vi "CleanGraph.vi"(9 "Bin Size":i32, 10 "N Sigma":dbl=4.0 format="%#_13g", 11 "XY Graph In":cluster{dbl[], dbl[]}(graph)) -> (3 "XY Graph Out":cluster{dbl[], dbl[]}(graph))   [LabVIEW 2019]
panel:
  in  "Repeat Until Clean (F: Run Once)":bool
  out "Smoothed":cluster{dbl[], dbl[]}(graph)
  out "Cleaned":cluster{dbl[], dbl[]}(graph)
  out "Ordered":cluster{dbl[], dbl[]}(graph)
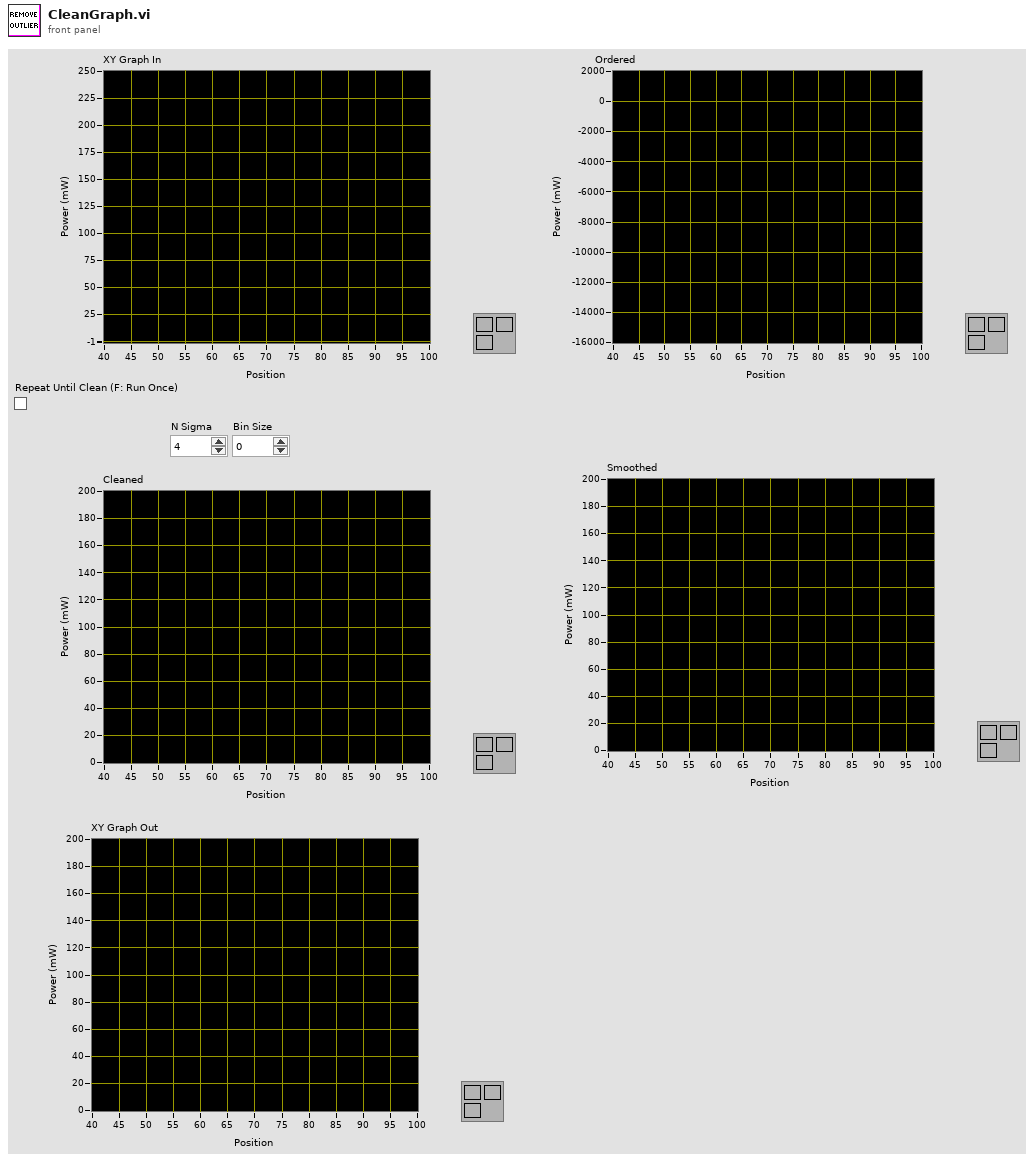
[diagram p1: front panel]
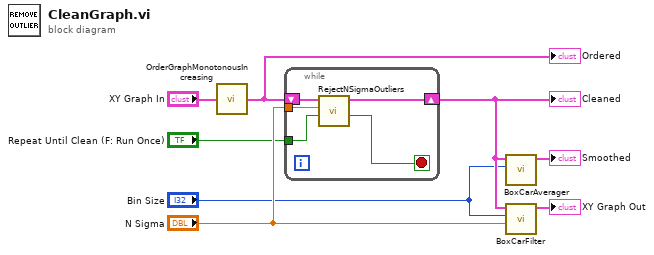
[diagram p0: block diagram]
diagram:
  n1 = call "OrderGraphMonotonousIncreasing.vi"("Power Graph"="XY Graph In") -> ("Cluster"=w6:cluster{dbl[], dbl[]})
  "Ordered" <- w6
  n2 = while {
    shift-right: [w13] -> w5
    shift-left: w6 -> [w12]
    tunnel: "N Sigma" -> [w10]
    tunnel: "Repeat Until Clean (F: Run Once)" -> [w9]
    stop <- w11 stop-if-true
    n3 = call "RejectNSigmaOutliers.vi"("Repeat Until Clean (F: Run Once)"=w9, "N Sigma"=w10, "Cluster in"=w12) -> ("Nothing Rejected"=w11:bool, "Cluster out"=w13:cluster{dbl[], dbl[]})  [unwired: 4 in, 3 out]
  }
  "Cleaned" <- w5
  n4 = call "BoxCarAverager.vi"("Bin Size"="Bin Size", "Graph in"=w5) -> ("Graph out"=→"Smoothed":cluster{dbl[], dbl[]})  [unwired: 7 in, 2 out]
  n5 = call "BoxCarFilter.vi"("N Sigma (3)"="N Sigma", "Bin Size (7)"="Bin Size", "Graph in"=w5) -> ("Graph out"=→"XY Graph Out":cluster{dbl[], dbl[]})  [unwired: 7 in, 1 out]
